vi "ManipulatePathsToINI.vi"(7 "BusIndex":i32, 8 "Error In":errorcluster, 11 "Bus in":refnum<class "Bus.lvclass">) -> (0 "Error Out":errorcluster, 3 "Bus out":refnum<class "Bus.lvclass">)   [LabVIEW 2018]
doc: "This VI manipulates the array of INI files to match the order of the PluginType listed in the Module array text ring."
uses:
  NistPluggableModules/BusClass/Bus.lvclass
  NistPluggableModules/BusClass/Bus.lvclass/Bus.ctl
  NistPluggableModules/TestClass/Test.lvclass/Test.ctl
  NistPluggableModules/TestClass/Accessors/Write PluginPathArray.vi
  NistPluggableModules/BusClass/Accessors/Read Test.vi
  NistPluggableModules/TestClass/Accessors/Read PluginPathArray.vi
  NistPluggableModules/BusClass/Accessors/Write Test.vi
  <vilib>/Utility/error.llb/Error Cluster From Error Code.vi
  NistPluggableModules/TestClass/Test.lvclass
  <vilib>/ErrorRing/Error Ring.xnode
panel:
  out "logical OR":bool
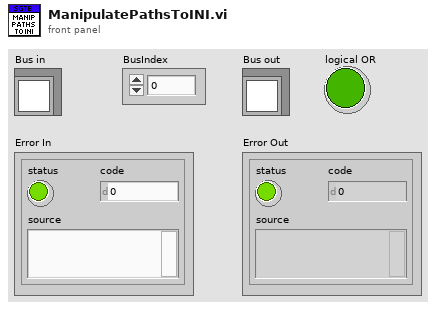
[diagram p1: front panel]
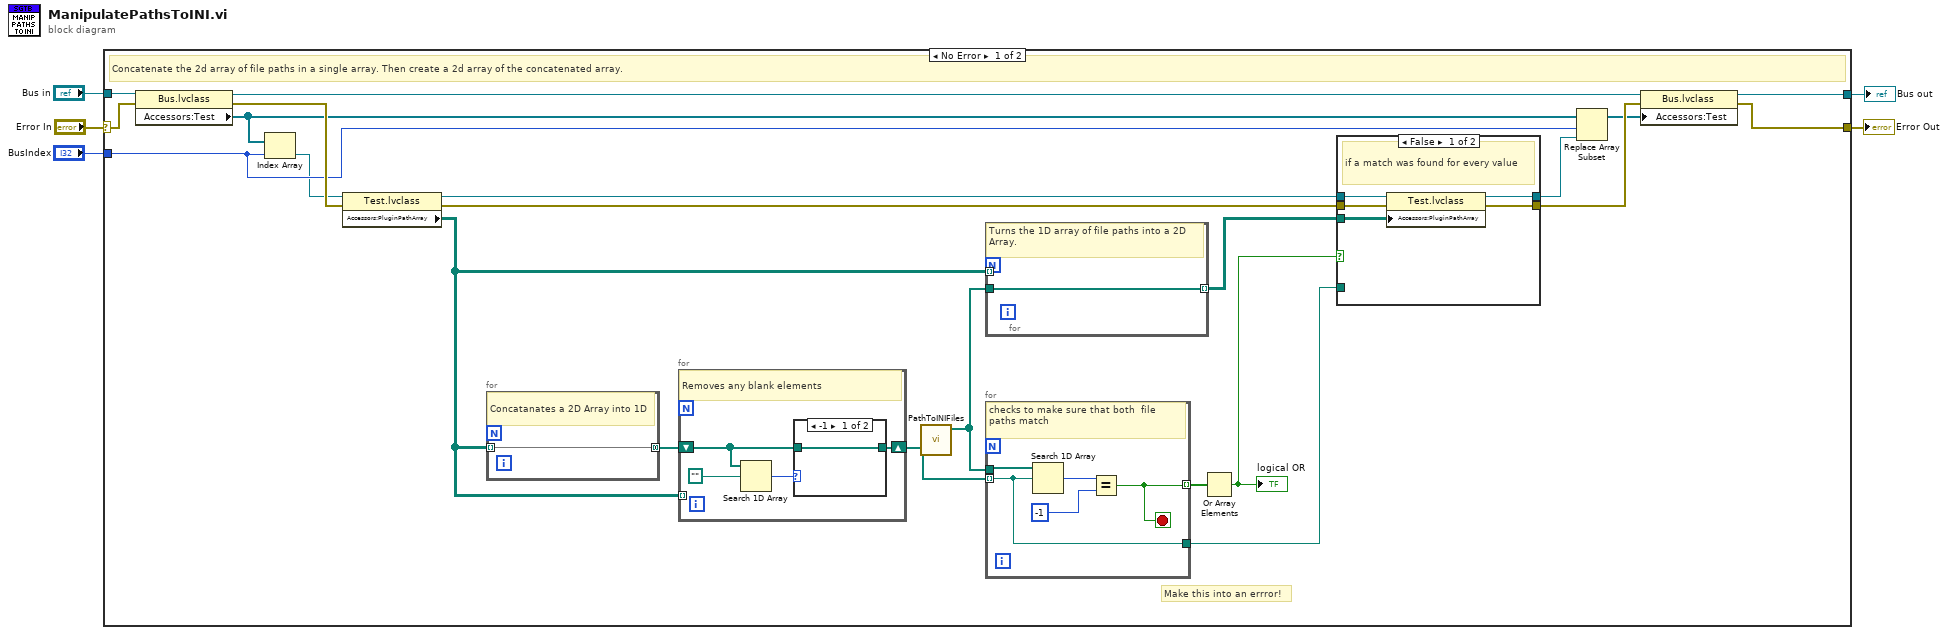
[diagram p0: block diagram]
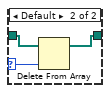
[diagram p2: hidden frame]
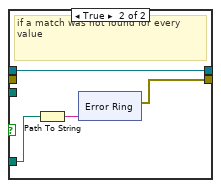
[diagram p3: hidden frame]
diagram:
  n1 = case shown="No Error" "Error In" {
    selector: "Error In" -> [w7 w59]
    tunnel: "Bus in" -> [w27 w60]
    tunnel: [w25 w60] -> w4
    tunnel: "BusIndex" -> [w19 _]
    tunnel: [w6 w59] -> w1
    frame No Error {
      # "Make this into an errror!"
      # "Concatenate the 2d array of file paths in a single array. Then create a 2d array of the concatenated array."
      n2 = property class="Bus.lvclass"(reference=w27, error in=w7) -> (reference out=w26:refnum<class "Bus.lvclass">, error out=w24:errorcluster, "Accessors:Test"=w17:refnum<class "Test.lvclass">[])
      n3 = Index Array(array=w17, index=w19) -> (element=w16:refnum<class "Test.lvclass">)
      n4 = property class="Test.lvclass"(reference=w16, error in=w24) -> (reference out=w23:refnum<class "Test.lvclass">, error out=w21:errorcluster, "Accessors:PluginPathArray"=w11:path[][])
      n5 = for {
        tunnel: w11 -> [w28] mode=indexing
        tunnel: [w28] -> w13 mode=concatenating
        # "Concatanates a 2D Array into 1D"
      }
      n6 = for {
        shift-right: [w32] -> w12
        shift-left: w13 -> [w31]
        tunnel: w11 -> [_] mode=indexing
        # "Removes any blank elements"
        n7 = Search 1D Array(1D array=w31, element=path "") -> (index of element=w30:i32)  [unwired: 1 in]
        n8 = case shown="-1" w30 {
          selector: w30 -> [_ w34]
          tunnel: w31 -> [w33 w36]
          tunnel: [w33 w35] -> w32
          frame -1 {
          }
          frame Default {
            n9 = Delete From Array(array=w36, index=w34) -> (array with subset deleted=w35:path[])  [unwired: 1 in, 1 out]
          }
        }
      }
      n10 = call "PathToINIFiles.vi"() -> ("IniFilePaths Out"=w14:path[])  [unwired: 11 in]
      n11 = for {
        tunnel: [w42] -> w15 mode=indexing
        tunnel: w14 -> [w42]
        tunnel: w11 -> [_] mode=indexing
        # "Turns the 1D array of file paths into a 2D Array."
      }
      n12 = for {
        tunnel: w12 -> [w37] mode=indexing
        tunnel: w14 -> [w41]
        tunnel: [w38] -> w9 mode=indexing
        tunnel: [w37] -> w10
        stop <- w38 stop-if-true
        # "checks to make sure that both  file paths match"
        n13 = Search 1D Array(1D array=w41, element=w37) -> (index of element=w40:i32)  [unwired: 1 in]
        n14 = Equal?(x=w40, y=-1) -> (x = y?=w38:bool)
      }
      n15 = Or Array Elements(Boolean array=w9) -> (logical OR=w8:bool)
      "logical OR" <- w8
      n16 = case shown="False" w8 {
        tunnel: w23 -> [w47 w51]
        tunnel: [w46 w50] -> w22
        tunnel: w21 -> [w45 _]
        tunnel: [w44 w51] -> w20
        tunnel: w15 -> [w43 _]
        tunnel: w10 -> [_ w49]
        frame False {
          # "if a match was found for every value"
          n17 = property class="Test.lvclass"(reference=w47, error in=w45, "Accessors:PluginPathArray"=w43) -> (reference out=w44:refnum<class "Test.lvclass">, error out=w46:errorcluster)
        }
        frame True {
          # "if a match was not found for every value"
          n18 = Path To String(path=w49) -> (string=w48:string)
          n19 = xnode "Error Ring"("parameter 0"=w48) -> ("error out"=w50:errorcluster)
        }
      }
      n20 = Replace Array Subset(array=w17, new element=w20, index=w19) -> (w18:refnum<class "Test.lvclass">[])
      n21 = property class="Bus.lvclass"(reference=w26, error in=w22, "Accessors:Test"=w18) -> (reference out=w25:refnum<class "Bus.lvclass">, error out=w6:errorcluster)
    }
    frame Error {
      # "If an error occurs passes the error through and does nothing."
    }
  }
  "Bus out" <- w4
  "Error Out" <- w1
